vi "PixyCam Loop.vi"   [LabVIEW 2016]
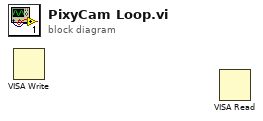
[diagram p0: block diagram]
diagram:
  n1 = VISA Write() -> ()  [unwired: 3 in, 3 out]
  n2 = VISA Read() -> ()  [unwired: 3 in, 4 out]
